vi "timeremaining.vi"(4 "endtime":string, 5 "starttime":string) -> (0 "time remaining":sgl format="%.2f", 1 "slot time":sgl format="%.2f", 2 "stop session":bool)   [LabVIEW 2010]
panel:
  out "seconds CURRENT":u32
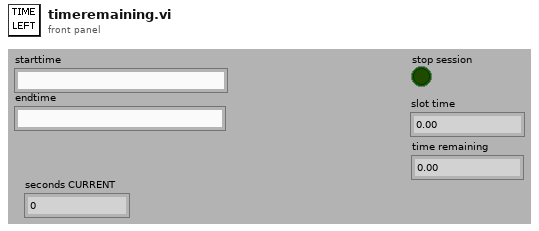
[diagram p1: front panel]
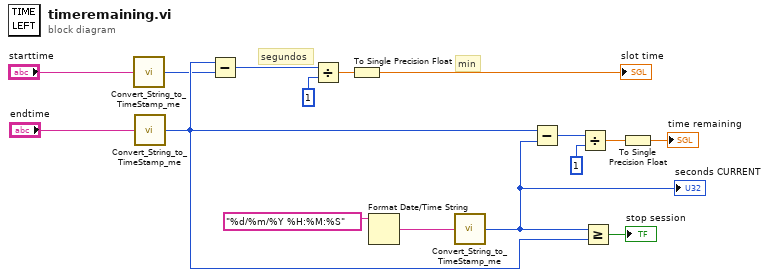
[diagram p0: block diagram]
diagram:
  # "min"
  # "segundos"
  n1 = call "Convert_String_to_TimeStamp_me.vi"("string timestamp"="starttime") -> ("seconds"=w1:u32)
  n2 = call "Convert_String_to_TimeStamp_me.vi"("string timestamp"="endtime") -> ("seconds"=w2:u32)
  n3 = Subtract(x=w2, y=w1) -> (x-y=w14:u32)
  n4 = Divide(x=w14, y=u32 1) -> (x/y=w12:dbl)
  n5 = To Single Precision Float(number=w12) -> (single precision float=→"slot time":sgl)
  n6 = Format Date/Time String(time format string (%c)="%d/%m/%Y %H:%M:%S") -> (date/time string=w11:string)  [unwired: 2 out]
  n7 = call "Convert_String_to_TimeStamp_me.vi"("string timestamp"=w11) -> ("seconds"=w6:u32)
  "seconds CURRENT" <- w6
  n8 = Subtract(x=w2, y=w6) -> (x-y=w9:u32)
  n9 = Divide(x=w9, y=u32 1) -> (x/y=w7:dbl)
  n10 = Greater Or Equal?(x=w6, y=w2) -> (x >= y?=→"stop session":bool)
  n11 = To Single Precision Float(number=w7) -> (single precision float=→"time remaining":sgl)
